vi "cv_02-02_subVI_thermometer.vi"() -> ()   [LabVIEW 2013]
panel:
  out "Thermometer":dbl(slide) scale=-58.0..212.0
  in  "stop":bool
  in  "Temp Scale":bool
  in  "Knob":dbl(knob) scale=-50.0..100.0
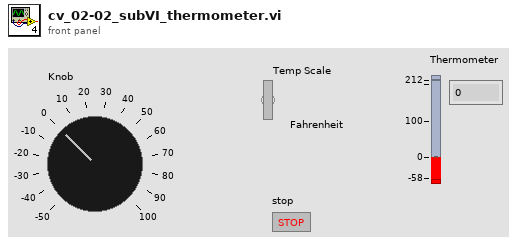
[diagram p1: front panel]
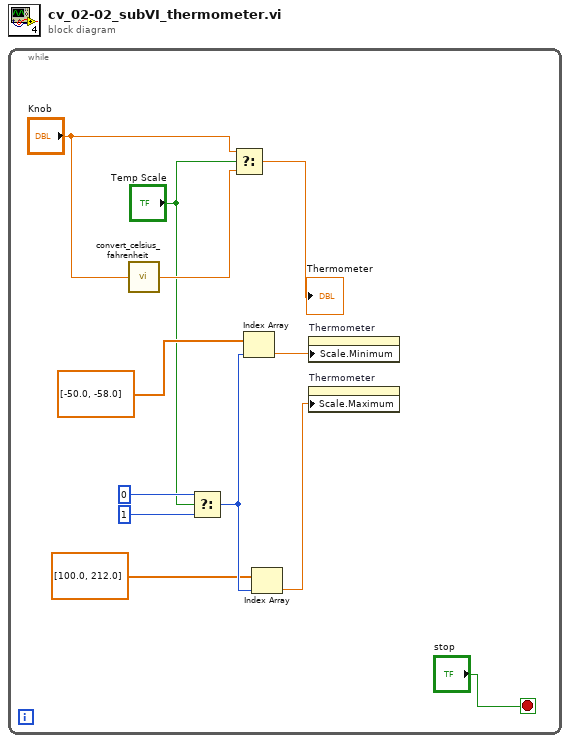
[diagram p0: block diagram]
diagram:
  n1 = while {
    stop <- "stop" stop-if-true
    n2 = call "convert_celsius_fahrenheit.vi"("Celsius"="Knob") -> ("Fahrenheit"=w9:dbl)
    n3 = Select(t=0, s="Temp Scale", f=1) -> (s? t:f=w3:i32)
    n4 = Select(t="Knob", s="Temp Scale", f=w9) -> (s? t:f=→"Thermometer":dbl)
    n5 = Index Array(array=dbl[] [-50.0, -58.0] ("Array"), index=w3) -> (element=w4:dbl)
    n6 = Index Array(array=dbl[] [100.0, 212.0] ("Array"), index=w3) -> (element=w1:dbl)
    n7 = property on="Thermometer" class="Slide (strict)"("Scale.Minimum"=w4) -> ()  [unwired: 2 in, 2 out]
    n8 = property on="Thermometer" class="Slide (strict)"("Scale.Maximum"=w1) -> ()  [unwired: 2 in, 2 out]
  }
